vi "Wave Generation - in time loop.vi"(0 "Pixel time (tick)":i32=80, 2 "Num of elements":u32=512000, 4 "Elements per line":i32=1000, 6 "Num of undershoot":i32=50, 7 "Resolution":i32=512, 8 "Pixel pulse_initial delay":i32=1, 9 "Pixel clock_pulse width(tick)":i32=40, 10 "Frame retrace time":u32=100 caption="Frame retrace time (ms)") -> (12 "Frame waveform output finish?":bool, 13 "Line clock":bool, 14 "Request address":u32, 16 "Galvo signal readed":u32, 17 "Data":u32, 19 "Pixel clock":bool)   [LabVIEW 2015]
doc: "nodes in time loop to avoid 10V jump"
uses:
  <vilib>/Platform/TimedLoop/XDataNode/timing_clust.ctl
  <vilib>/Platform/TimedLoop/XDataNode/nitl_modes.ctl
  <vilib>/Platform/TimedLoop/XDataNode/wakeup.ctl
  DRAM data index.ctl
  <vilib>/rvi/eio/common/nirviEmuTemplateMethod_errors.vi
  <vilib>/rvi/Emulation/niFpgaSctlEmulationGetInTimedLoop.vi
  <vilib>/rvi/Emulation/niFpgaEmulationReportErrorSimple.vi
  <vilib>/rvi/Emulation/niFpgaGetClockAttributes.vi
  <vilib>/rvi/Emulation/niFpgaCriticalErrorInLSC.vi
  <vilib>/rvi/Emulation/niFpgaProcessEmulError.vi
  <vilib>/eio/EIONode/EIONode.xnode
  <vilib>/Platform/TimedLoop/XDataNode/XDataNode.xnode
  <vilib>/Platform/TimedLoop/XDataNode/XDNodeRunTimeDep.lvlib
  Globals/Global_Sample per Frame.vi
panel:
  out "Numeric":i32
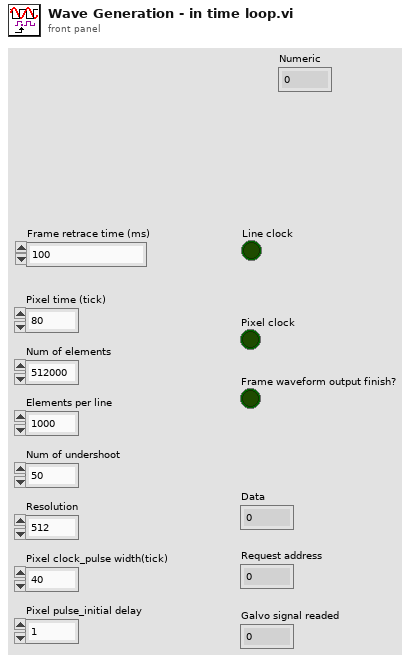
[diagram p1: front panel]
types:
  T1 = typedef "XDNodeRunTimeDep.lvlib/timing_clust.ctl" = cluster{"Expected End [f-1]":u64, "Actual End [f-1]":u64, "Finished Late? [f-1]":bool, "Expected End [i-1]":u64, "Actual End [i-1]":u64, "Finished Late? [i-1]":bool, "Expected Start [i]":u64, "Actual Start [i]":u64, "Expected Start [f]":u64, "Actual Start [f]":u64, "Source Name":string, "Structure Name":string, "Period":i64, "Deadline":i64, "Offset":i64, "Start":i64, "Priority":i32, "Timeout":i32, "Mode":T2, "Wakeup Reason":T3, "Error":errorcluster, "Source Type":string, "Secondary Source Type":string, "Global End Time":u64, "Global Start Time":u64, "Frame Duration":u64, "Iteration Duration":u64, "Assigned CPU":i32, "I/O Scan Engine Mode":u32}
  T2 = typedef "XDNodeRunTimeDep.lvlib/nitl_modes.ctl" = enum32{"No Change", "Process missed periods, maintain original phase", "Discard missed periods, maintain original phase", "Process missed periods, ignore original phase", "Discard missed periods, ignore original phase"}
  T3 = typedef "XDNodeRunTimeDep.lvlib/wakeup.ctl" = enum32{"Normal", "Aborted", "Asynchronous wakeup", "Timing source error", "Timed loop error", "Timeout"}
  T4 = typedef "DRAM data index.ctl" = enum16{"Numeric 1", "Numeric 2", "Numeric 3", "Numeric 4", "Numeric 5", "Numeric 6", "Numeric 7", "Numeric 8", "Numeric 9", "Numeric 10", "Numeric 11", "Numeric 12", "Numeric 13", "Numeric 14", "Numeric 15", "Numeric 16"}
  T5 = cluster{"Numeric 1":u32, "Numeric 2":u32, "Numeric 3":u32, "Numeric 4":u32, "Numeric 5":u32, "Numeric 6":u32, "Numeric 7":u32, "Numeric 8":u32, "Numeric 9":u32, "Numeric 10":u32, "Numeric 11":u32, "Numeric 12":u32, "Numeric 13":u32, "Numeric 14":u32, "Numeric 15":u32, "Numeric 16":u32}
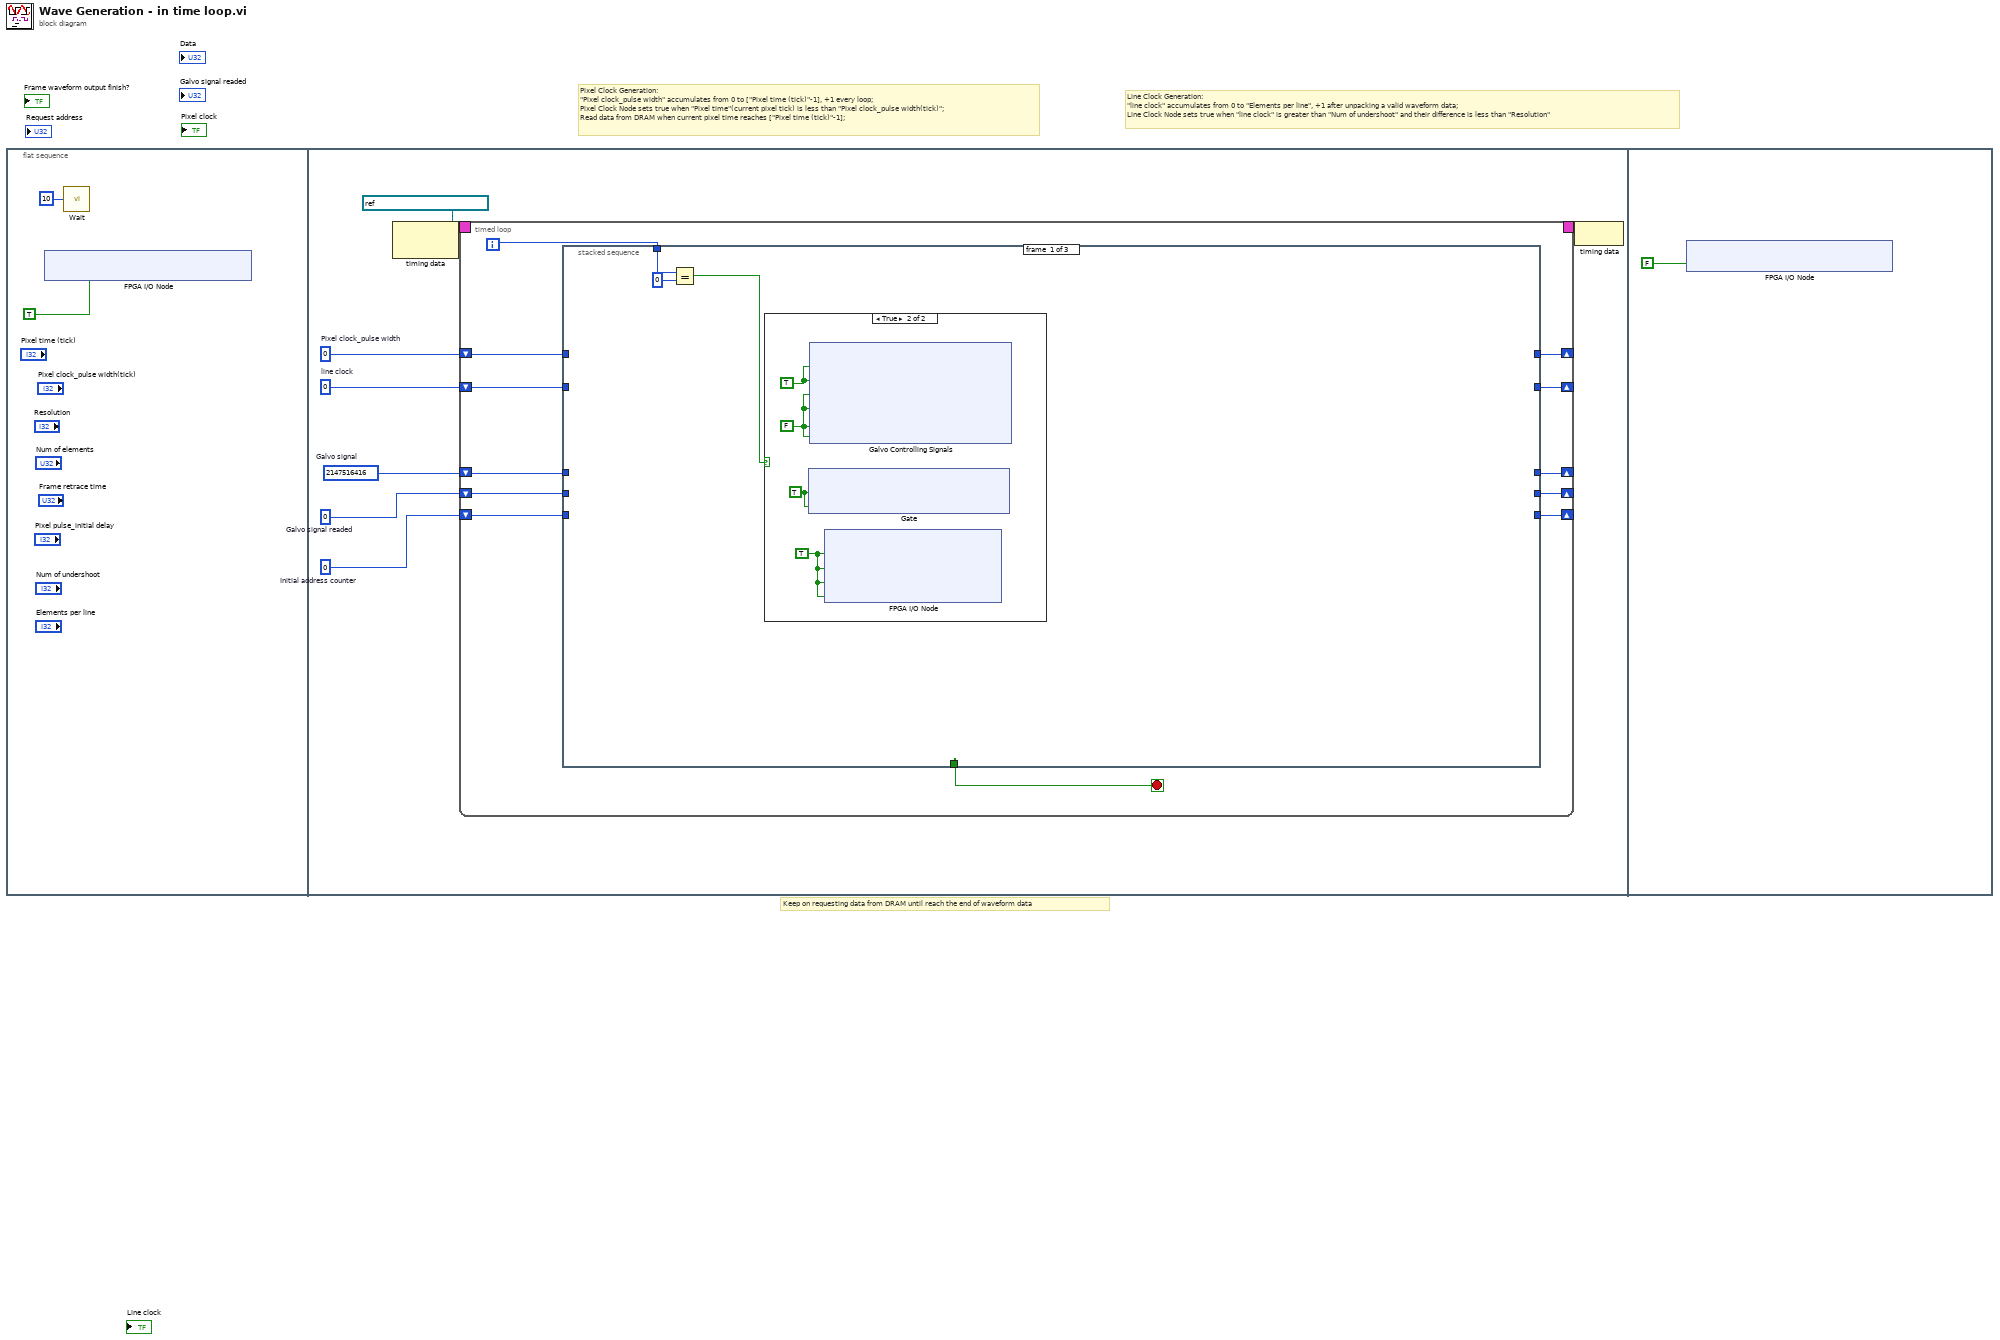
[diagram p0: block diagram]
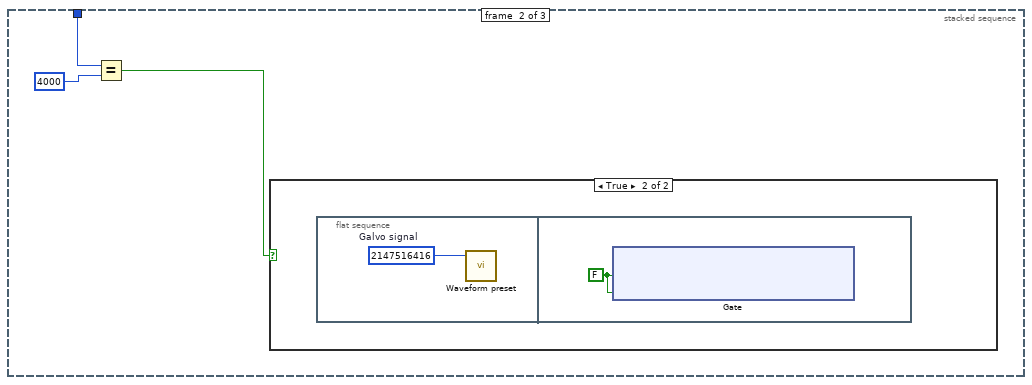
[diagram p3: hidden frame]
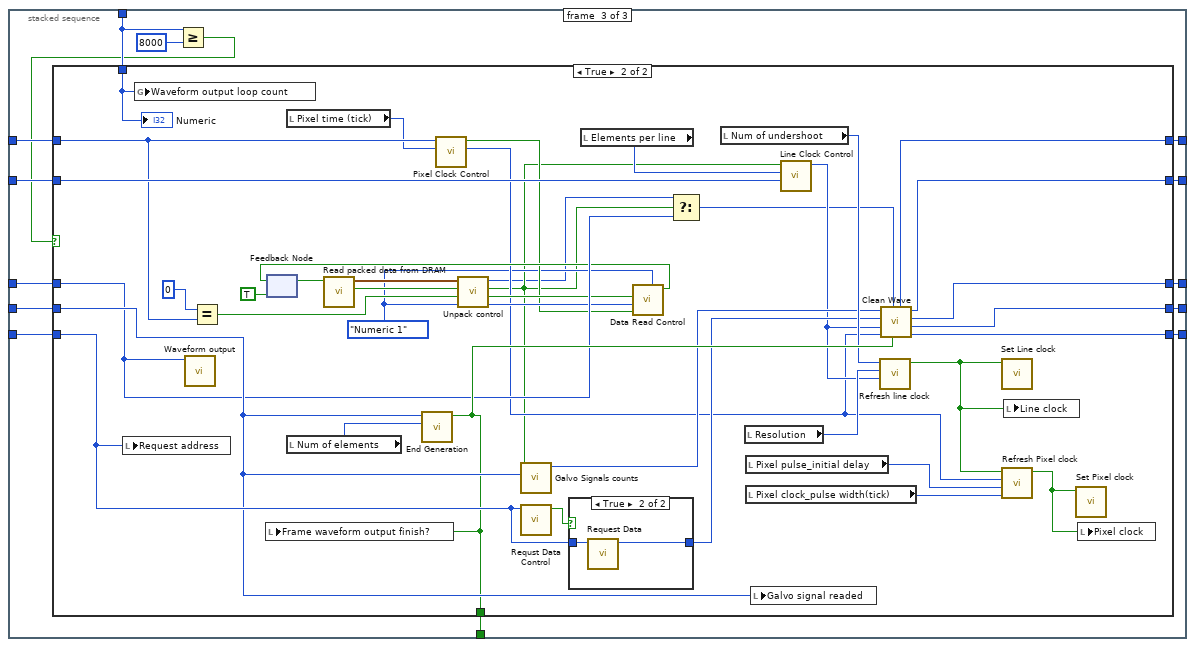
[diagram p5: hidden frame]
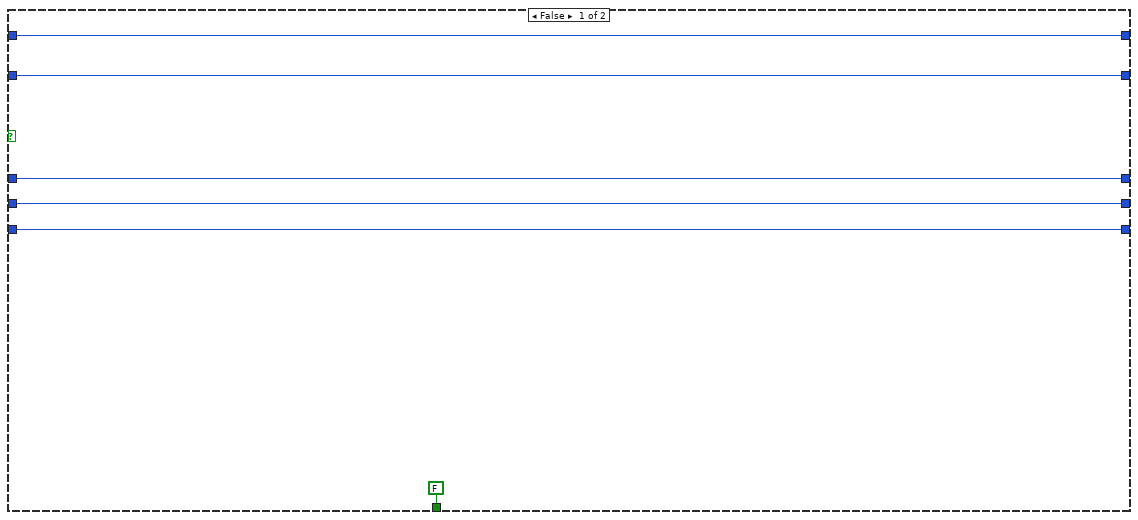
[diagram p6: hidden frame]
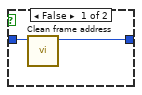
[diagram p7: hidden frame]
diagram:
  # "Keep on requesting data from DRAM until reach the end of waveform data"
  # "Line Clock Generation:\n\"line clock\" accumulates from 0 to \"Elements per line\", +1 after unpacking a valid waveform data;\nLine Clock Node sets true when \"line clock\" is greater than \"Num of undershoot\" and their difference is less than \"Resolution\""
  # "Pixel Clock Generation: \n\"Pixel clock_pulse width\" accumulates from 0 to [\"Pixel time (tick)\"-1], +1 every loop;\nPixel Clock Node sets true when \"Pixel time\"(current pixel tick) is less than \"Pixel clock_pulse width(tick)\";\nRead data from DRAM when current pixel time reaches [\"Pixel time (tick)\"-1];"
  n1 = flat-sequence {
    frame #0 {
      n2 = xnode "FPGA I/O Node"("IO Module\\Shutter(DDCA_PFI1_WRITE)"=TRUE ("IO Module\\Shutter(DDCA_PFI1_WRITE)")) -> ()  [unwired: 1 in, 1 out]
      n3 = call "Wait"("Count(uSec)"=u32 10) -> ()  [unwired: 1 out]
    }
    frame #1 {
      w7 = u32 0  # Initial address counter
      w4 = 0  # Pixel clock_pulse width
      w5 = 0  # line clock
      w6 = u32 0  # Galvo signal readed
      w3 = u32 2147516416  # Galvo signal
      n4 = node-c288(refnum<k21> "40 MHz Onboard Clock" ("Source Name")) -> (w10:T1)
      n5 = timed-loop {
        timing: w10 -> [_]
        timing-out: [_] -> w9
        shift-right: [w15] -> _
        shift-left: w7 -> [w21]
        shift-right: [w18] -> _
        shift-left: w3 -> [w13]
        shift-right: [w17] -> _
        shift-left: w6 -> [w19]
        shift-right: [w16] -> _
        shift-left: w5 -> [w22]
        shift-right: [w12] -> _
        shift-left: w4 -> [w20]
        i -> [w11]
        stop <- w14 stop-if-true
        n6 = stacked-sequence {
          tunnel: w22 -> [_ _ w48]
          tunnel: w21 -> [_ _ w47]
          tunnel: w20 -> [_ _ w46]
          tunnel: w19 -> [_ _ w45]
          tunnel: [_ _ w44] -> w18
          tunnel: [_ _ w43] -> w17
          tunnel: [_ _ w42] -> w16
          tunnel: [_ _ w41] -> w15
          tunnel: [_ _ w40] -> w14
          tunnel: w13 -> [_ _ w39]
          tunnel: [_ _ w38] -> w12
          tunnel: w11 -> [w25 w32 w37]
          frame #0 {
            n7 = Equal?(x=w25, y=0) -> (x = y?=w23:bool)
            n8 = case shown="True" w23 {
              frame False {
              }
              frame True {
                w26 = TRUE ("IO Module\\DDCA_DIO8-15_WE")
                w27 = TRUE ("IO Module\\LDAx(DDCB_DIO6_WRITE)")
                w28 = FALSE ("_CSx")
                w29 = TRUE ("_CLRx")
                n9 = xnode "Gate"("IO Module\\LDAx(DDCB_DIO6_WRITE)"=w27, "IO Module\\LDAy(DDCB_DIO7_WRITE)"=w27) -> ()  [unwired: 2 in, 2 out]
                n10 = xnode "Galvo Controlling Signals"("IO Module\\CLRx(DDCB_DIO0_WRITE)"=w29, "IO Module\\CLRy(DDCB_DIO1_WRITE)"=w29, "IO Module\\CSx(DDCB_DIO2_WRITE)"=w28, "IO Module\\CSy(DDCB_DIO3_WRITE)"=w28, "IO Module\\R_Wx(DDCB_DIO4_WRITE)"=w28, "IO Module\\R_Wy(DDCB_DIO5_WRITE)"=w28) -> ()  [unwired: 6 in, 6 out]
                n11 = xnode "FPGA I/O Node"("IO Module\\DDCA_DIO8-15_WE"=w26, "IO Module\\DDCA_DIO16-23_WE"=w26, "IO Module\\DDCB_DIO8-15_WE"=w26, "IO Module\\DDCB_DIO16-23_WE"=w26) -> ()  [unwired: 4 in, 4 out]
              }
            }
          }
          frame #1 {
            n12 = Equal?(x=w32, y=4000) -> (x = y?=w30:bool)
            n13 = case shown="True" w30 {
              frame False {
              }
              frame True {
                n14 = flat-sequence {
                  frame #0 {
                    w33 = u32 2147516416  # Galvo signal
                    n15 = call "Waveform preset.vi"("Galvo signal"=w33) -> ()  [unwired: 11 in]
                  }
                  frame #1 {
                    w34 = FALSE ("IO Module\\LDAx(DDCB_DIO6_WRITE)")
                    n16 = xnode "Gate"("IO Module\\LDAx(DDCB_DIO6_WRITE)"=w34, "IO Module\\LDAy(DDCB_DIO7_WRITE)"=w34) -> ()  [unwired: 2 in, 2 out]
                  }
                }
              }
            }
          }
          frame #2 {
            n17 = Greater Or Equal?(x=w37, y=8000) -> (x >= y?=w35:bool)
            n18 = case shown="True" w35 {
              tunnel: w48 -> [w53 w94]
              tunnel: w47 -> [w50 w93]
              tunnel: w46 -> [w54 w92]
              tunnel: w45 -> [w51 w91]
              tunnel: [w52 w90] -> w44
              tunnel: [w51 w89] -> w43
              tunnel: [w53 w88] -> w42
              tunnel: [w50 w87] -> w41
              tunnel: [FALSE ("End Generation") w86] -> w40
              tunnel: w39 -> [w52 w85]
              tunnel: [w54 w84] -> w38
              tunnel: w37 -> [_ w55]
              frame False {
              }
              frame True {
                w59 = DRAM_data_index."Numeric 1" ("DRAM pack index out")
                n19 = local write "Request address"(w93) -> ()
                n20 = global write "Global_Sample per Frame.vi" "Waveform output loop count"(w55) -> ()
                n21 = call "Waveform output.vi"("Galvo signal"=w85) -> ()  [unwired: 11 in]
                n22 = Equal?(x=0, y=w92) -> (x = y?=w76:bool)
                n23 = feedback #1(TRUE) -> (w78:bool)
                n24 = local read "Pixel time (tick)"() -> (w75:i32)
                n25 = local read "Num of elements"() -> (w71:u32)
                n26 = call "Read packed data from DRAM.vi"("Output ready"=w78) -> ("Output Valid§"=w82:bool, "Data"=w81:T5)  [unwired: 9 in]
                n27 = call "End Generation.vi"("Num of elements"=w71, "Galvo signal readed"=w91) -> ("End Generation"=w86:bool)  [unwired: 9 in]
                n28 = local write "Frame waveform output finish?"(w86) -> ()
                n29 = call "Pixel Clock Control.vi"("Pixel time (tick)"=w75, "Pixel clock_pulse width"=w92) -> ("Pixel time"=w61:i32, "Pixel time up"=w60:bool)  [unwired: 8 in]
                n30 = call "Unpack control.vi"("DRAM pack index init"=w59, "enable unpack"=w76, "input valid"=w82, "Data"=w81) -> ("output valid?"=w74:bool, "output valid? 2"=w58:bool, "Unpacked data"=w57:u32, "DRAM pack index out out"=w72:T4)  [unwired: 4 in]
                n31 = call "Galvo Signals counts.vi"("Galvo signal readed in"=w91, "output valid? in"=w58) -> ("Galvo signal readed out"=w64:u32)  [unwired: 9 in]
                n32 = call "Requst Data Control.vi"("Initial address counter"=w93) -> ("Enable request"=w79:bool)  [unwired: 10 in]
                n33 = case shown="True" w79 {
                  tunnel: w93 -> [w95 w98]
                  tunnel: [w96 w97] -> w63
                  frame False {
                    n34 = call "Clean frame address.vi"("Initial address counter in"=w95) -> ("Initial address counter out"=w96:u32)  [unwired: 10 in]
                  }
                  frame True {
                    n35 = call "Request Data.vi"("Address counter"=w98) -> ("Address counter output"=w97:u32)  [unwired: 10 in]
                  }
                }
                n36 = local read "Elements per line"() -> (w83:i32)
                n37 = call "Data Read Control.vi"("DRAM pack index out"=w59, "Pixel time up"=w60, "DRAM pack index out out"=w72, "input valid?"=w74) -> ("output valid"=w73:bool)  [unwired: 7 in]
                n38 = feedback-in #1(w73) -> ()
                n39 = Select(t=w57, s=w58, f=w85) -> (s? t:f=w56:u32)
                n40 = local read "Num of undershoot"() -> (w69:i32)
                n41 = local read "Resolution"() -> (w70:i32)
                n42 = local read "Pixel pulse_initial delay"() -> (w67:i32)
                n43 = local read "Pixel clock_pulse width(tick)"() -> (w66:i32)
                n44 = local write "Galvo signal readed"(w91) -> ()
                n45 = call "Line Clock Control.vi"("line clock in"=w94, "Elements per line"=w83, "output valid? in"=w58) -> ("line clock out"=w62:i32)  [unwired: 8 in]
                n46 = call "Refresh line clock.vi"("line clock output"=w62, "Resolution"=w70, "Num of undershoot"=w69) -> ("Refresh?"=w68:bool)  [unwired: 8 in]
                n47 = call "Clean Wave.vi"("line clock out"=w62, "Galvo signal in"=w56, "pixel clock_pulse width in"=w61, "Clean wave"=w86, "Address counter output"=w63, "Galvo signal readed out"=w64) -> ("Address counter"=w87:u32, "Galvo signal readed out"=w89:u32, "Galvo signal in"=w90:u32, "line clock"=w88:i32, "pixel clock_pulse width out"=w84:i32)  [unwired: 1 in]
                n48 = call "Set Line clock.vi"("Refresh"=w68) -> ()  [unwired: 11 in]
                n49 = call "Refresh Pixel clock.vi"("Pixel clock_pulse width(tick)"=w66, "Pixel pulse_initial delay"=w67, "Pixel clock_pulse width"=w61, "Refresh input"=w68) -> ("Refresh output"=w65:bool)  [unwired: 7 in]
                n50 = local write "Line clock"(w68) -> ()
                n51 = call "Set Pixel clock.vi"("Refresh"=w65) -> ()  [unwired: 11 in]
                n52 = local write "Pixel clock"(w65) -> ()
                "Numeric" <- w55
              }
            }
          }
        }
      }
      n53 = node-c288(w9) -> ()
    }
    frame #2 {
      n54 = xnode "FPGA I/O Node"("IO Module\\Shutter(DDCA_PFI1_WRITE)"=FALSE ("IO Module\\Shutter(DDCA_PFI1_WRITE)")) -> ()  [unwired: 1 in, 1 out]
    }
  }
